vi "Digitizer Voltage AutoScale.vi"(2 "Card Type":enum16{"DP 110", "DP 310"}(ring), 3 "Vert Scale Lookup Table":sgl[](array[numeric]), 4 "Main Digitizer":u16, 5 "NI Card":refnum<k15>, 6 "Positive Peak":dbl, 7 "Negitive Peak":dbl, 8 "Channel":i32=1, 9 "Acq Card ID":u32, 10 "Vert Settings In":cluster{sgl, i32, "Coupling":u16}) -> (0 "Vert Settings Out":cluster{sgl, i32, "Coupling":u16}, 1 "Success?":bool)   [LabVIEW 2022 SP3]
panel:
  in  "Threshold":dbl=1.1
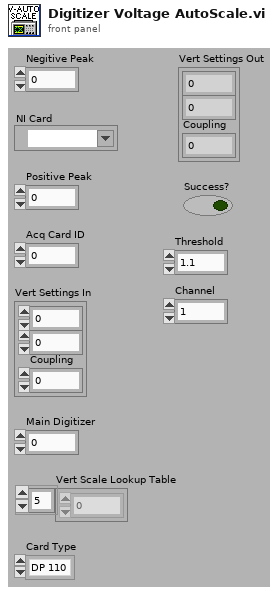
[diagram p1: front panel]
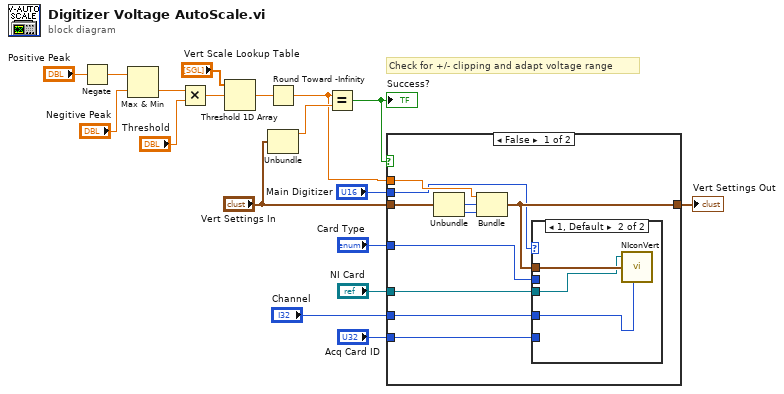
[diagram p0: block diagram]
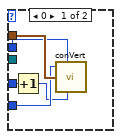
[diagram p2: hidden frame]
diagram:
  # "Check for +/- clipping and adapt voltage range"
  n1 = Negate(x="Positive Peak") -> (-x=w3:dbl)
  n2 = Max & Min(x=w3, y="Negitive Peak") -> (min(x,y)=w5:dbl)  [unwired: 1 out]
  n3 = Multiply(x=w5, y="Threshold") -> (x*y=w4:dbl)
  n4 = Threshold 1D Array(2:w4, 3:"Vert Scale Lookup Table") -> (0:w8:sgl)  [unwired: 1 out]
  n5 = Round Toward -Infinity(1:w8) -> (0:w1:sgl)
  n6 = Unbundle("Vert Settings In") -> (w7:sgl)  [unwired: 2 out]
  n7 = Equal?(x=w1, y=w7) -> (x = y?=w16:bool)
  "Success?" <- w16
  n8 = case shown="False" w16 {
    tunnel: [w24 w37] -> w17
    tunnel: "Vert Settings In" -> [w26 w37]
    tunnel: w1 -> [w25 _]
    tunnel: "Card Type" -> [w23 _]
    tunnel: "Acq Card ID" -> [w22 _]
    tunnel: "Main Digitizer" -> [w21 _]
    tunnel: "NI Card" -> [w20 _]
    tunnel: "Channel" -> [w19 _]
    frame False {
      n9 = Unbundle(w26) -> (w28:i32, "Coupling"=w27:u16)  [unwired: 1 out]
      n10 = Bundle(w25, w28, "Coupling"=w27) -> (w24:cluster{sgl, i32, "Coupling":u16})  [unwired: 1 out]
      n11 = case shown="1, Default" w21 {
        tunnel: w24 -> [w33 w36]
        tunnel: w23 -> [w32 _]
        tunnel: w22 -> [w31 _]
        tunnel: w20 -> [_ w35]
        tunnel: w19 -> [w30 w34]
        frame 0 {
          n12 = Increment(x=w30) -> (x+1=w29:i32)
          n13 = call "conVert.vi"("InstrumentID"=w31, 1:w32, "V scale"=w33, "Channel (1)"=w29) -> ()  [unwired: 1 in, 3 out]
        }
        frame 1, Default {
          n14 = call "NIconVert.vi"("InstrumentID"=w35, "V scale"=w36, "Channel (0)"=w34) -> ()  [unwired: 1 in, 4 out]
        }
      }
    }
    frame True {
    }
  }
  "Vert Settings Out" <- w17
